vi "Edit Data.vi"(8 "error in (no error)":errorcluster, 10 "All Data":refnum<class "Data Item.lvclass">[](array[class]), 11 "Data Item in":refnum<class "Data Item.lvclass">) -> (0 "error out":errorcluster, 1 "OK?":bool, 2 "All Data out":refnum<class "Data Item.lvclass">[](array[class]), 3 "Data Item out":refnum<class "Data Item.lvclass">)   [LabVIEW 2026, in "VILab.lvlib" / "Data Item.lvclass"]
uses:
  Data Item.lvclass
  Data Item.lvclass/Data Item.ctl
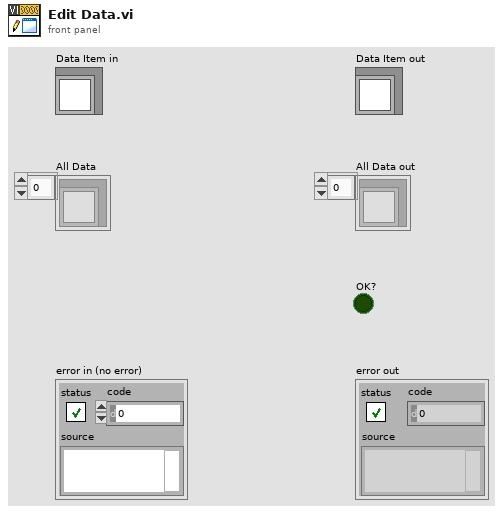
[diagram p1: front panel]
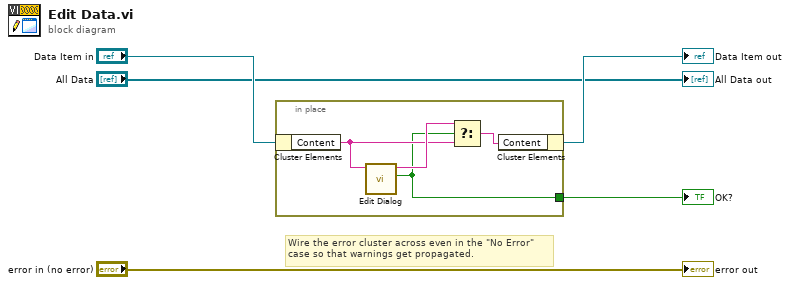
[diagram p0: block diagram]
diagram:
  # "Wire the error cluster across even in the \"No Error\"\ncase so that warnings get propagated."
  n1 = in-place {
    in-place-border: [w6] -> w1
    n2 = in-place-cluster #1("Data Item in") -> ("Content"=w7:string)
    n3 = call "Edit Dialog.vi"("Content"=w7) -> ("OK?"=w6:bool, "String"=w9:string)  [unwired: 9 in]
    n4 = Select(t=w9, s=w6, f=w7) -> (s? t:f=w8:string)
    n5 = in-place-cluster #1("Content"=w8) -> (→"Data Item out":refnum<class "Data Item.lvclass">)
  }
  "OK?" <- w1
  "error out" <- "error in (no error)"
  "All Data out" <- "All Data"
